vi "S2C_PCIe1762H_Proc_Commands.vi"(7 "VI_Ref":refnum<vi>, 8 "Error In":errorcluster, 10 "Settings":T1, 11 "Q-Ref":refnum<queue>) -> (0 "Error Out":errorcluster, 2 "Stop?":bool, 3 "Response":variant)   [LabVIEW 2024]
uses:
  S2C_PCIe1762H_Proc_Globals.vi
  _Shared/S2C_Shared_Proc_Globals.vi
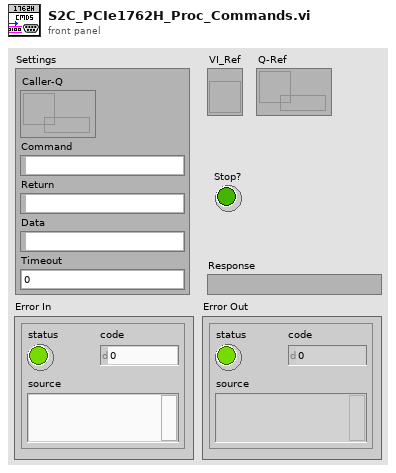
[diagram p1: front panel]
types:
  T1 = cluster{"Caller-Q":refnum<queue>, "Command":string, "Return":string, "Data":variant, "Timeout":dbl}
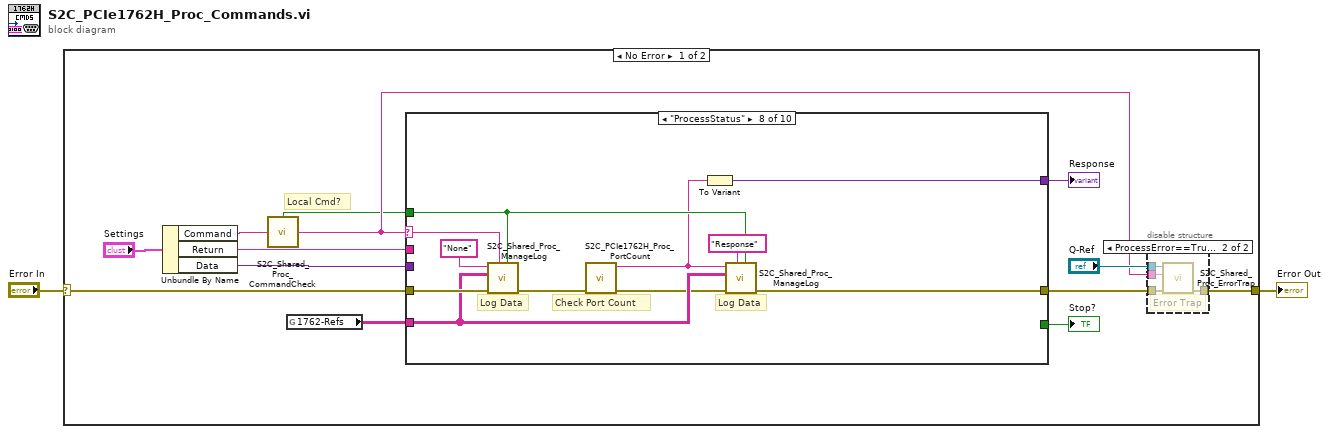
[diagram p0: block diagram]
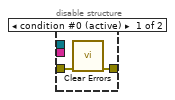
[diagram p2: hidden frame]
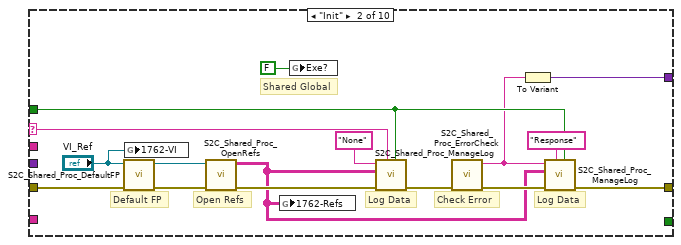
[diagram p4: hidden frame]
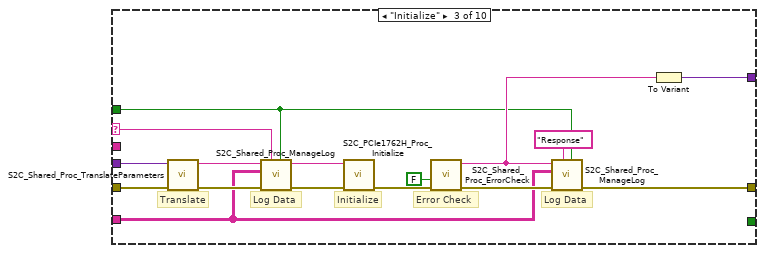
[diagram p5: hidden frame]
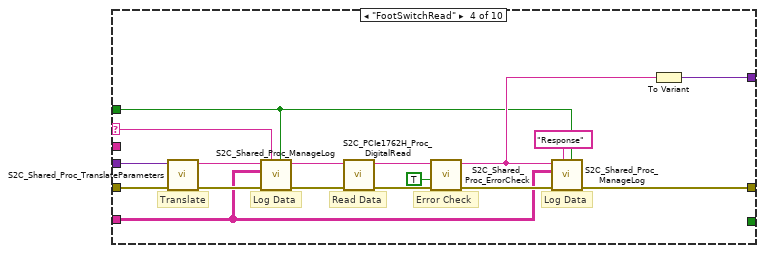
[diagram p6: hidden frame]
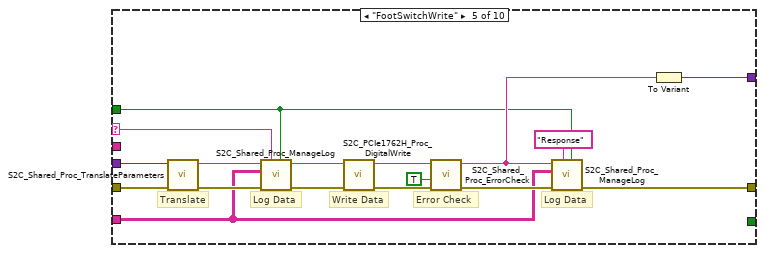
[diagram p7: hidden frame]
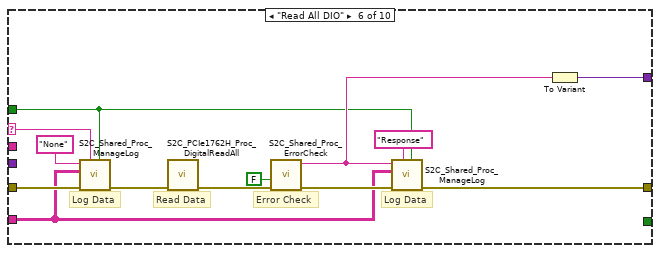
[diagram p8: hidden frame]
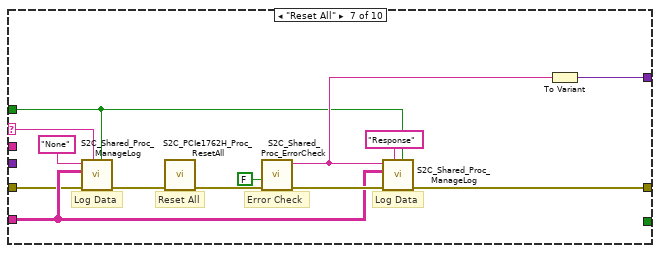
[diagram p9: hidden frame]
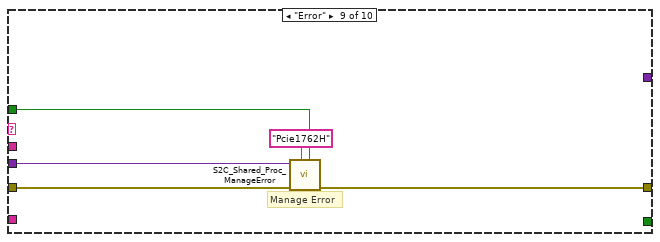
[diagram p10: hidden frame]
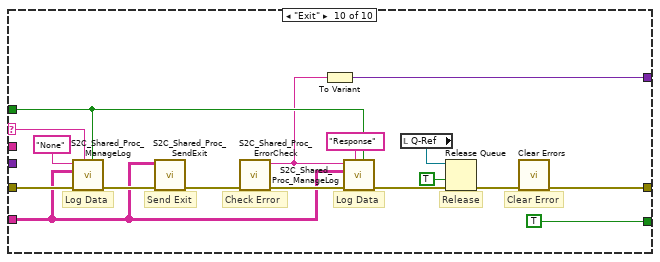
[diagram p11: hidden frame]
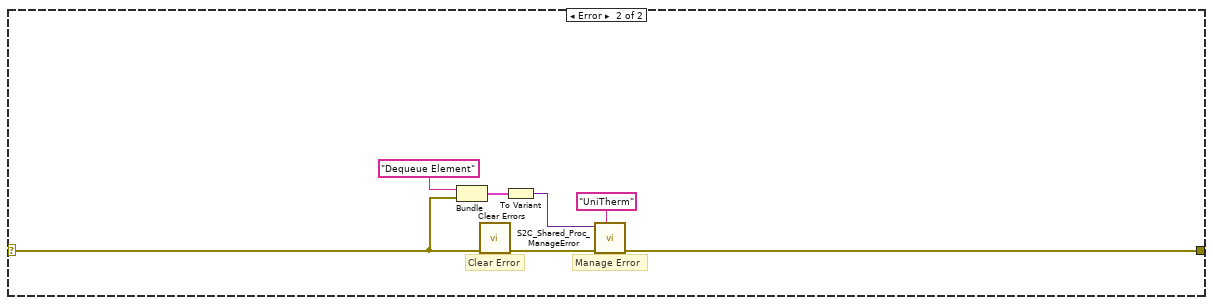
[diagram p12: hidden frame]
diagram:
  n1 = case shown="No Error" "Error In" {
    selector: "Error In" -> [w14 w151]
    tunnel: [w7 w153] -> w1
    frame No Error {
      # "Local Cmd?"
      n2 = Unbundle By Name("Settings") -> ("Command"=w6:string, "Return"=w10:string, "Data"=w15:variant)
      n3 = call "S2C_Shared_Proc_CommandCheck.vi"("Cmd In"=w6) -> ("Local?"=w4:bool, "Cmd Out"=w5:string)  [unwired: 13 in]
      n4 = global read "S2C_PCIe1762H_Proc_Globals.vi" "1762-Refs"() -> (w3:string[][])
      n5 = case shown="\"ProcessStatus\"" w5 {
        selector: w5 -> [_ w35 w45 w60 w77 w93 w105 w124 _ w144]
        tunnel: w14 -> [w22 w27 w43 w58 w75 w94 w106 w123 w129 w145]
        tunnel: w15 -> [_ _ w44 w59 w76 _ _ _ w126 _]
        tunnel: [w22 w38 w41 w56 w73 w96 w108 w120 w128 w132] -> w8
        tunnel: [_ w32 w40 w55 w72 w95 w107 w121 _ w139] -> w12
        tunnel: [_ _ _ _ _ _ _ _ _ TRUE] -> w11
        tunnel: w10 -> [_ _ _ _ _ _ _ _ _ _]
        tunnel: w4 -> [_ w36 w46 w61 w78 w92 w104 w118 w127 w143]
        tunnel: w3 -> [_ _ w42 w57 w74 w91 w109 w119 _ w136]
        frame "Other", Default {
        }
        frame "Init" {
          # "Default FP"
          # "Shared Global"
          # "Check Error"
          # "Log Data"
          # "Open Refs"
          # "Log Data"
          n6 = call "S2C_Shared_Proc_DefaultFP.vi"("Error In"=w27, "VI_Ref In"="VI_Ref") -> ("Error Out"=w25:errorcluster, "VI_Ref Out"=w26:refnum<vi>)  [unwired: 8 in]
          n7 = global write "S2C_PCIe1762H_Proc_Globals.vi" "1762-VI"("VI_Ref") -> ()
          n8 = call "S2C_Shared_Proc_OpenRefs.vi"("Error In"=w25, "VI_Ref"=w26) -> ("Error Out"=w28:errorcluster, "Refs"=w24:string[][])  [unwired: 8 in]
          n9 = global write "S2C_PCIe1762H_Proc_Globals.vi" "1762-Refs"(w24) -> ()
          n10 = global write "S2C_Shared_Proc_Globals.vi" "Exe?"(FALSE ("Exe?")) -> ()
          n11 = call "S2C_Shared_Proc_ManageLog.vi"("Local?"=w36, "Command"=w35, "Error In"=w28, "Refs"=w24, "Data In"="None") -> ("Error Out"=w30:errorcluster)  [unwired: 5 in, 1 out]
          n12 = call "S2C_Shared_Proc_ErrorCheck.vi"("Error In"=w30) -> ("Error Out"=w33:errorcluster, "Status"=w31:string)  [unwired: 9 in]
          n13 = To Variant(anything=w31) -> (Variant=w32:variant)
          n14 = call "S2C_Shared_Proc_ManageLog.vi"("Local?"=w36, "Command"="Response", "Error In"=w33, "Refs"=w24, "Data In"=w31) -> ("Error Out"=w38:errorcluster)  [unwired: 5 in, 1 out]
        }
        frame "Initialize" {
          # "Initialize"
          # "Error Check"
          # "Log Data"
          # "Log Data"
          # "Translate"
          n15 = call "S2C_Shared_Proc_TranslateParameters.vi"("Error In"=w43, "Data"=w44) -> ("Error Out"=w53:errorcluster, "JSON Cluster"=w54:string)  [unwired: 8 in]
          n16 = call "S2C_Shared_Proc_ManageLog.vi"("Local?"=w46, "Command"=w45, "Error In"=w53, "Refs"=w42, "Data In"=w54) -> ("Error Out"=w52:errorcluster, "Data Out"=w39:string)  [unwired: 5 in]
          n17 = call "S2C_PCIe1762H_Proc_Initialize.vi"("Error In"=w52, "Initialize"=w39) -> ("Error Out"=w49:errorcluster)  [unwired: 9 in]
          n18 = call "S2C_Shared_Proc_ErrorCheck.vi"("Error In"=w49, "ExpReply?"=FALSE) -> ("Error Out"=w50:errorcluster, "Status"=w48:string)  [unwired: 8 in]
          n19 = call "S2C_Shared_Proc_ManageLog.vi"("Local?"=w46, "Command"="Response", "Error In"=w50, "Refs"=w42, "Data In"=w48) -> ("Error Out"=w41:errorcluster)  [unwired: 5 in, 1 out]
          n20 = To Variant(anything=w48) -> (Variant=w40:variant)
        }
        frame "FootSwitchRead" {
          # "Read Data"
          # "Error Check"
          # "Log Data"
          # "Log Data"
          # "Translate"
          n21 = call "S2C_Shared_Proc_TranslateParameters.vi"("Error In"=w58, "Data"=w59) -> ("Error Out"=w70:errorcluster, "JSON Cluster"=w71:string)  [unwired: 8 in]
          n22 = call "S2C_Shared_Proc_ManageLog.vi"("Local?"=w61, "Command"=w60, "Error In"=w70, "Refs"=w57, "Data In"=w71) -> ("Error Out"=w68:errorcluster, "Data Out"=w69:string)  [unwired: 5 in]
          n23 = call "S2C_PCIe1762H_Proc_DigitalRead.vi"("Error In"=w68, "FootSwitch"=w69) -> ("Error Out"=w65:errorcluster, "Result"=w63:string)  [unwired: 8 in]
          n24 = call "S2C_Shared_Proc_ErrorCheck.vi"("Error In"=w65, "ExpReply?"=TRUE, "Reply Text"=w63) -> ("Error Out"=w66:errorcluster, "Status"=w64:string)  [unwired: 7 in]
          n25 = call "S2C_Shared_Proc_ManageLog.vi"("Local?"=w61, "Command"="Response", "Error In"=w66, "Refs"=w57, "Data In"=w64) -> ("Error Out"=w56:errorcluster)  [unwired: 5 in, 1 out]
          n26 = To Variant(anything=w64) -> (Variant=w55:variant)
        }
        frame "FootSwitchWrite" {
          # "Write Data"
          # "Error Check"
          # "Log Data"
          # "Log Data"
          # "Translate"
          n27 = call "S2C_Shared_Proc_TranslateParameters.vi"("Error In"=w75, "Data"=w76) -> ("Error Out"=w87:errorcluster, "JSON Cluster"=w88:string)  [unwired: 8 in]
          n28 = call "S2C_Shared_Proc_ManageLog.vi"("Local?"=w78, "Command"=w77, "Error In"=w87, "Refs"=w74, "Data In"=w88) -> ("Error Out"=w85:errorcluster, "Data Out"=w86:string)  [unwired: 5 in]
          n29 = call "S2C_PCIe1762H_Proc_DigitalWrite.vi"("Error In"=w85, "FootSwitch"=w86) -> ("Error Out"=w82:errorcluster, "Result"=w80:string)  [unwired: 8 in]
          n30 = call "S2C_Shared_Proc_ErrorCheck.vi"("Error In"=w82, "ExpReply?"=TRUE, "Reply Text"=w80) -> ("Error Out"=w83:errorcluster, "Status"=w81:string)  [unwired: 7 in]
          n31 = call "S2C_Shared_Proc_ManageLog.vi"("Local?"=w78, "Command"="Response", "Error In"=w83, "Refs"=w74, "Data In"=w81) -> ("Error Out"=w73:errorcluster)  [unwired: 5 in, 1 out]
          n32 = To Variant(anything=w81) -> (Variant=w72:variant)
        }
        frame "Read All DIO" {
          # "Read Data"
          # "Error Check"
          # "Log Data"
          # "Log Data"
          n33 = call "S2C_Shared_Proc_ManageLog.vi"("Local?"=w92, "Command"=w93, "Error In"=w94, "Refs"=w91, "Data In"="None") -> ("Error Out"=w101:errorcluster)  [unwired: 5 in, 1 out]
          n34 = call "S2C_PCIe1762H_Proc_DigitalReadAll.vi"("Error In"=w101) -> ("Error Out"=w89:errorcluster)  [unwired: 10 in]
          n35 = call "S2C_Shared_Proc_ErrorCheck.vi"("Error In"=w89, "ExpReply?"=FALSE) -> ("Error Out"=w99:errorcluster, "Status"=w98:string)  [unwired: 8 in]
          n36 = call "S2C_Shared_Proc_ManageLog.vi"("Local?"=w92, "Command"="Response", "Error In"=w99, "Refs"=w91, "Data In"=w98) -> ("Error Out"=w96:errorcluster)  [unwired: 5 in, 1 out]
          n37 = To Variant(anything=w98) -> (Variant=w95:variant)
        }
        frame "Reset All" {
          # "Reset All"
          # "Error Check"
          # "Log Data"
          # "Log Data"
          n38 = call "S2C_Shared_Proc_ManageLog.vi"("Local?"=w104, "Command"=w105, "Error In"=w106, "Refs"=w109, "Data In"="None") -> ("Error Out"=w114:errorcluster)  [unwired: 5 in, 1 out]
          n39 = call "S2C_PCIe1762H_Proc_ResetAll.vi"("Error In"=w114) -> ("Error Out"=w103:errorcluster)  [unwired: 10 in]
          n40 = call "S2C_Shared_Proc_ErrorCheck.vi"("Error In"=w103, "ExpReply?"=FALSE) -> ("Error Out"=w112:errorcluster, "Status"=w111:string)  [unwired: 8 in]
          n41 = call "S2C_Shared_Proc_ManageLog.vi"("Local?"=w104, "Command"="Response", "Error In"=w112, "Refs"=w109, "Data In"=w111) -> ("Error Out"=w108:errorcluster)  [unwired: 5 in, 1 out]
          n42 = To Variant(anything=w111) -> (Variant=w107:variant)
        }
        frame "ProcessStatus" {
          # "Check Port Count"
          # "Log Data"
          # "Log Data"
          n43 = call "S2C_Shared_Proc_ManageLog.vi"("Local?"=w118, "Command"=w124, "Error In"=w123, "Refs"=w119, "Data In"="None") -> ("Error Out"=w117:errorcluster)  [unwired: 5 in, 1 out]
          n44 = call "S2C_PCIe1762H_Proc_PortCount.vi"("Error In"=w117) -> ("Error Out"=w116:errorcluster, "Result"=w115:string)  [unwired: 9 in]
          n45 = To Variant(anything=w115) -> (Variant=w121:variant)
          n46 = call "S2C_Shared_Proc_ManageLog.vi"("Local?"=w118, "Command"="Response", "Error In"=w116, "Refs"=w119, "Data In"=w115) -> ("Error Out"=w120:errorcluster)  [unwired: 5 in, 1 out]
        }
        frame "Error" {
          # "Manage Error"
          n47 = call "S2C_Shared_Proc_ManageError.vi"("Local?"=w127, "Process"="Pcie1762H", "Error In"=w129, "Data"=w126) -> ("Error Out"=w128:errorcluster)  [unwired: 7 in]
        }
        frame "Exit" {
          # "Clear Error"
          # "Release"
          # "Check Error"
          # "Send Exit"
          # "Log Data"
          # "Log Data"
          n48 = call "S2C_Shared_Proc_ManageLog.vi"("Local?"=w143, "Command"=w144, "Error In"=w145, "Refs"=w136, "Data In"="None") -> ("Error Out"=w137:errorcluster)  [unwired: 5 in, 1 out]
          n49 = call "S2C_Shared_Proc_SendExit.vi"("Error In"=w137, "Refs"=w136) -> ("Error Out"=w131:errorcluster)  [unwired: 9 in]
          n50 = call "S2C_Shared_Proc_ErrorCheck.vi"("Error In"=w131) -> ("Error Out"=w141:errorcluster, "Status"=w138:string)  [unwired: 9 in]
          n51 = To Variant(anything=w138) -> (Variant=w139:variant)
          n52 = call "S2C_Shared_Proc_ManageLog.vi"("Local?"=w143, "Command"="Response", "Error In"=w141, "Refs"=w136, "Data In"=w138) -> ("Error Out"=w140:errorcluster)  [unwired: 5 in, 1 out]
          n53 = local read "Q-Ref"() -> (w134:refnum<queue>)
          n54 = Release Queue(queue=w134, force destroy? (F)=TRUE, error in (no error)=w140) -> (error out=w135:errorcluster)  [unwired: 2 out]
          n55 = call <vilib>:"Clear Errors.vi"("error in (no error)"=w135) -> ("error out"=w132:errorcluster)  [unwired: 5 in, 1 out]
        }
      }
      "Response" <- w12
      "Stop?" <- w11
      n56 = disable-structure shown="ProcessError==True" {
        disable-tunnel: w8 -> [w17 w21]
        disable-tunnel: [w16 w20] -> w7
        disable-tunnel: w5 -> [_ w19]
        disable-tunnel: "Q-Ref" -> [_ w18]
        frame condition #0 (active) {
          n57 = call <vilib>:"Clear Errors.vi"("error in (no error)"=w17) -> ("error out"=w16:errorcluster)  [unwired: 5 in, 1 out]
        }
        frame condition #1 {
          # "Error Trap"
          n58 = call "S2C_Shared_Proc_ErrorTrap.vi"("Error In"=w21, "Command"=w19, "Q-Ref"=w18) -> ("Error Out"=w20:errorcluster)  [unwired: 8 in]
        }
      }
    }
    frame Error {
      # "Clear Error"
      # "Manage Error"
      n59 = Bundle("Dequeue Element", "error IO"=w151) -> (w152:cluster{string, "error IO":errorcluster})  [unwired: 1 in]
      n60 = call <vilib>:"Clear Errors.vi"("error in (no error)"=w151) -> ("error out"=w148:errorcluster)  [unwired: 5 in, 1 out]
      n61 = To Variant(anything=w152) -> (Variant=w149:variant)
      n62 = call "S2C_Shared_Proc_ManageError.vi"("Process"="UniTherm", "Error In"=w148, "Data"=w149) -> ("Error Out"=w153:errorcluster)  [unwired: 8 in]
    }
  }
  "Error Out" <- w1
